vi "GEOM_VAR_DataBasePath.vi"(9 "Action":T1, 10 "Path":path) -> (2 "GEOM_coordsref out":path)   [LabVIEW 2016]
uses:
  GEOM_VAR_action.ctl
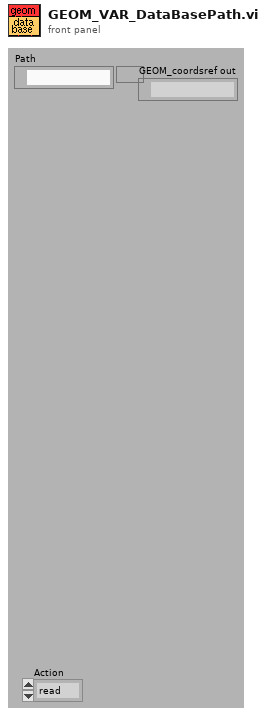
[diagram p1: front panel]
types:
  T1 = typedef "GEOM_VAR_action.ctl" = enum16{"read", "write"}
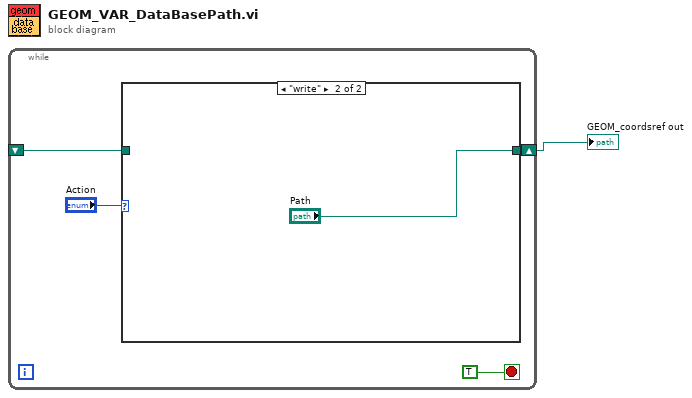
[diagram p0: block diagram]
diagram:
  n1 = while {
    shift-right: [w2] -> w1
    shift-left: _ -> [w4]
    stop <- TRUE stop-if-true
    n2 = case shown="\"write\"" "Action" {
      tunnel: w4 -> [w6 _]
      tunnel: [w6 "Path"] -> w2
      frame "read", Default {
      }
      frame "write" {
      }
    }
  }
  "GEOM_coordsref out" <- w1
